vi "controlContinousFwd.vi"(7 "Set":bool, 8 "error in":errorcluster, 9 "continous FWD in":bool=TRUE, 10 "axis in":u8, 11 "connection ID":refnum<k5>) -> (0 "error out":errorcluster, 1 "continous FWD out":bool=TRUE, 2 "axis out":u8, 3 "connection ID":refnum<k5>)   [LabVIEW 2019]
panel:
  in  "Set Command":string="com.attocube.amc.move.setControlContinousFwd"
  in  "Get Command":string="com.attocube.amc.move.getControlContinousFwd"
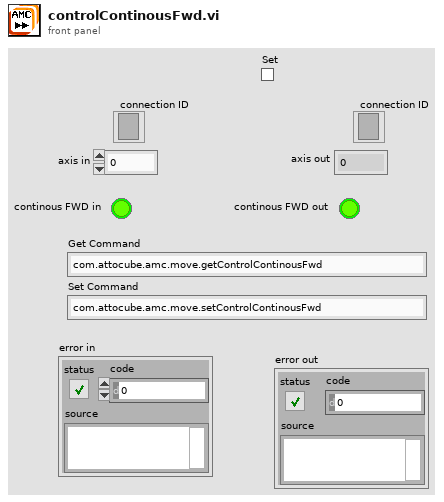
[diagram p1: front panel]
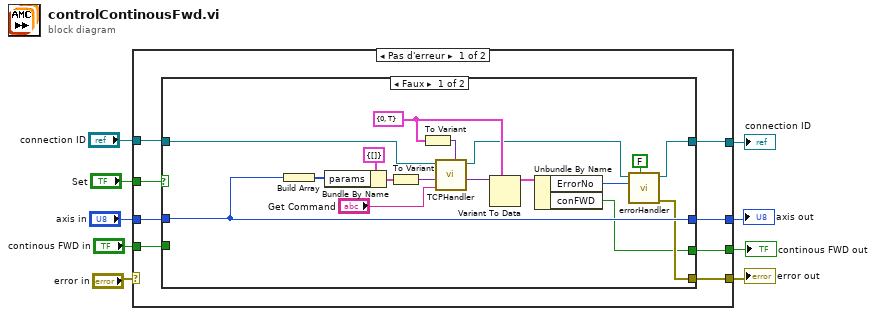
[diagram p0: block diagram]
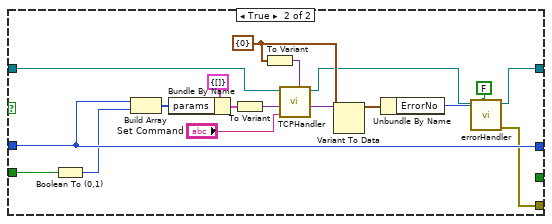
[diagram p2: hidden frame]
diagram:
  n1 = case shown="Pas d'erreur" "error in" {
    selector: "error in" -> [_ w56]
    tunnel: "axis in" -> [w14 w54]
    tunnel: [w10 w56] -> w8
    tunnel: [w12 w54] -> w7
    tunnel: "Set" -> [w16 _]
    tunnel: [w11 w55] -> w5
    tunnel: "continous FWD in" -> [w15 w55]
    tunnel: [w13 w53] -> w3
    tunnel: "connection ID" -> [w17 w53]
    frame No Error {
      n2 = case shown="Faux" w16 {
        tunnel: [w18 w35] -> w13
        tunnel: w17 -> [w24 w47]
        tunnel: w14 -> [w26 w45]
        tunnel: [w26 w45] -> w12
        tunnel: [w23 _] -> w11
        tunnel: [w25 w42] -> w10
        tunnel: w15 -> [_ w38]
        frame False {
          w21 = cluster{"ErrorNo":i16, "conFWD":bool} {"ErrorNo"=0, "conFWD"=TRUE} ("input cluster")
          n3 = Build Array(w26) -> (w30:u8[])
          n4 = Bundle By Name(cluster=cluster{"params":i16[]} {"params"=[]} ("input cluster"), "params"=w30) -> (w31:cluster{"params":i16[]})
          n5 = To Variant(anything=w31) -> (Variant=w32:variant)
          n6 = To Variant(anything=w21) -> (Variant=w22:variant)
          n7 = call "TCPHandler.vi"("result Types"=w22, "method"="Get Command", "params"=w32, "connection ID"=w24) -> ("result"=w28:variant, "connection ID"=w19:refnum<k5>)  [unwired: 5 in, 1 out]
          n8 = Variant To Data(type=w21, Variant=w28) -> (data=w33:cluster{"ErrorNo":i16, "conFWD":bool})  [unwired: 1 in, 1 out]
          n9 = Unbundle By Name(w33) -> ("ErrorNo"=w34:i16, "conFWD"=w23:bool)
          n10 = call "errorHandler.vi"("show popup"=FALSE, "error number"=w34, "connection ID"=w19) -> ("error out"=w25:errorcluster, "connection ID"=w18:refnum<k5>)  [unwired: 7 in]
        }
        frame True {
          w40 = cluster{"ErrorNo":i16} {"ErrorNo"=0} ("input cluster")
          n11 = Boolean To (0,1)(Boolean=w38) -> (0, 1=w39:i16)
          n12 = Build Array(w45, w39) -> (w49:i16[])
          n13 = Bundle By Name(cluster=cluster{"params":i64[]} {"params"=[]} ("input cluster"), "params"=w49) -> (w48:cluster{"params":i64[]})
          n14 = To Variant(anything=w48) -> (Variant=w46:variant)
          n15 = To Variant(anything=w40) -> (Variant=w41:variant)
          n16 = call "TCPHandler.vi"("result Types"=w41, "method"="Set Command", "params"=w46, "connection ID"=w47) -> ("result"=w51:variant, "connection ID"=w36:refnum<k5>)  [unwired: 5 in, 1 out]
          n17 = Variant To Data(type=w40, Variant=w51) -> (data=w44:cluster{"ErrorNo":i16})  [unwired: 1 in, 1 out]
          n18 = Unbundle By Name(w44) -> ("ErrorNo"=w43:i16)
          n19 = call "errorHandler.vi"("show popup"=FALSE, "error number"=w43, "connection ID"=w36) -> ("error out"=w42:errorcluster, "connection ID"=w35:refnum<k5>)  [unwired: 7 in]
        }
      }
    }
    frame Error {
    }
  }
  "error out" <- w8
  "axis out" <- w7
  "continous FWD out" <- w5
  "connection ID" <- w3
